vi "Cleanup (User).vi"(8 "error in":errorcluster, 11 "Node in":refnum<class "AMS Climate Chamber Template.lvclass">) -> (0 "error out":errorcluster caption="error in", 3 "Node out":refnum<class "AMS Climate Chamber Template.lvclass">)   [LabVIEW 2023, in "AMS Climate Chamber Template.lvlib" / "AMS Climate Chamber Template.lvclass"]
uses:
  AMS Climate Chamber Template.lvclass
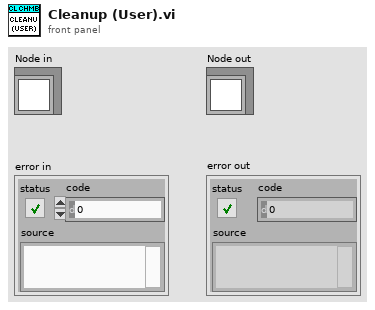
[diagram p1: front panel]
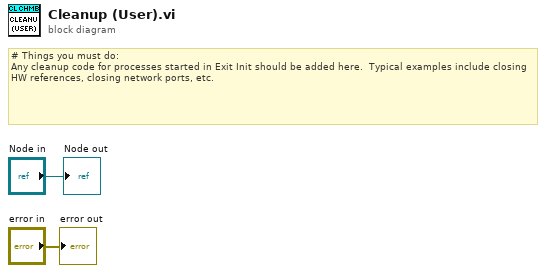
[diagram p0: block diagram]
diagram:
  # "# Things you must do:\nAny cleanup code for processes started in Exit Init should be added here.  Typical examples include closing HW references, closing network ports, etc."
  "Node out" <- "Node in"
  "error out" <- "error in"
